vi "TCP Check - Server.vi"() -> ()   [LabVIEW 2020]
panel:
  in  "Client Closed":string="The client VI closed the connection."
  in  "Stop":bool
  out "Waveform Graph":u8[](graph)
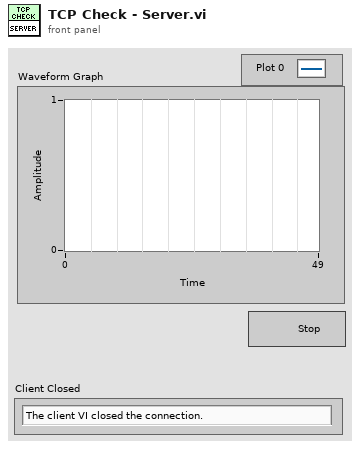
[diagram p1: front panel]
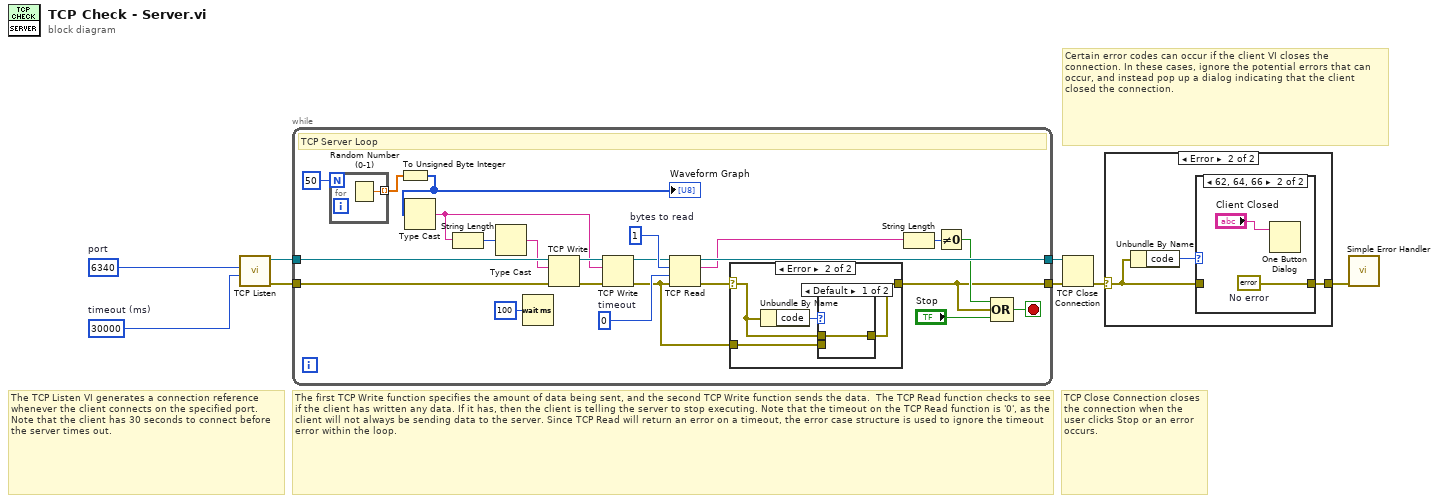
[diagram p0: block diagram]
diagram:
  w1 = u16 6340  # port
  w2 = 30000  # timeout (ms)
  # "TCP Close Connection closes the connection when the user clicks Stop or an error occurs."
  # "The TCP Listen VI generates a connection reference whenever the client connects on the specified port. Note that the client has 30 seconds to connect before the server times out."
  # "Certain error codes can occur if the client VI closes the connection. In these cases, ignore the potential errors that can occur, and instead pop up a dialog indicating that the client closed the connection."
  # "The first TCP Write function specifies the amount of data being sent, and the second TCP Write function sends the data.  The TCP Read function checks to see if the client has written any data. If it has, then the client is telling the server to stop executing. Note that the timeout on the TCP Read function is '0', as the client will not always be sending data to the server. Since TCP Read will return an error on a timeout, the error case structure is used to ignore the timeout error within the loop."
  n1 = call <vilib>:"TCP Listen.vi"("timeout ms (wait forever: -1)"=w2, "port"=w1) -> ("error out"=w3:errorcluster, "connection ID"=w4:refnum<k5>)  [unwired: 5 in, 3 out]
  n2 = while {
    tunnel: [w12] -> w7
    tunnel: [w18] -> w8
    tunnel: w4 -> [w31]
    tunnel: w3 -> [w22]
    stop <- w24 stop-if-true
    w17 = 0  # timeout
    w20 = 1  # bytes to read
    # "TCP Server Loop"
    n3 = for {
      N: 50 ("# of Points") -> [_]
      tunnel: [w39] -> w10 mode=indexing
      n4 = Random Number (0-1)() -> (number: 0 to 1=w39:dbl)
    }
    n5 = To Unsigned Byte Integer(number=w10) -> (unsigned 8bit integer=w9:u8[])
    "Waveform Graph" <- w9
    n6 = Type Cast(x=w9) -> (*(type *) &x=w26:string)  [unwired: 1 out]
    n7 = String Length(string=w26) -> (length=w28:i32)
    n8 = Type Cast(x=w28) -> (*(type *) &x=w27:string)  [unwired: 1 out]
    n9 = Wait (ms)(milliseconds to wait=u32 100) -> ()  [unwired: 1 out]
    n10 = TCP Write(connection ID=w31, data in=w27, error in (no error)=w22) -> (connection ID out=w30:refnum<k5>, error out=w29:errorcluster)  [unwired: 2 out]
    n11 = TCP Write(connection ID=w30, data in=w26, error in (no error)=w29) -> (connection ID out=w19:refnum<k5>, error out=w11:errorcluster)  [unwired: 2 out]
    n12 = TCP Read(connection ID=w19, bytes to read=w20, error in (no error)=w11, 9:w17) -> (connection ID out=w18:refnum<k5>, data out=w15:string, error out=w13:errorcluster)  [unwired: 1 out]
    n13 = case shown="Error" w13 {
      selector: w13 -> [w32 w35]
      tunnel: [w32 w33] -> w12
      tunnel: w11 -> [_ w34]
      frame No Error {
      }
      frame Error {
        n14 = Unbundle By Name(w35) -> ("code"=w36:i32)
        n15 = case shown="Default" w36 {
          tunnel: w35 -> [w37 _]
          tunnel: w34 -> [_ w38]
          tunnel: [w37 w38] -> w33
          frame Default {
          }
          frame 56 {
          }
        }
      }
    }
    n16 = String Length(string=w15) -> (length=w16:i32)
    n17 = Not Equal To 0?(x=w16) -> (x != 0?=w14:bool)
    n18 = Compound Arithmetic op=OR(w14, w12, "Stop") -> (w24:bool)
  }
  n19 = TCP Close Connection(connection ID=w8, error in (no error)=w7) -> (error out=w6:errorcluster)  [unwired: 2 out]
  n20 = case shown="Error" w6 {
    selector: w6 -> [w40 w42]
    tunnel: [w40 w41] -> w5
    frame No Error {
    }
    frame Error {
      n21 = Unbundle By Name(w42) -> ("code"=w43:i32)
      n22 = case shown="62, 64, 66" w43 {
        tunnel: w42 -> [w44 _]
        tunnel: [w44 w46] -> w41
        frame Default {
        }
        frame 62, 64, 66 {
          w46 = errorcluster {"status"=FALSE, "code"=0, "source"=""}  # No error
          n23 = One Button Dialog(message="Client Closed") -> ()  [unwired: 1 in, 1 out]
        }
      }
    }
  }
  n24 = call <vilib>:"Simple Error Handler.vi"("error in (no error)"=w5) -> ()  [unwired: 1 in, 8 out]
